vi "Check_Aero_Tunnel_on_Server.vi"(0 "Values":dbl[](array[numeric]) format="%.2f", 2 "Ch Names":string[](array[string]), 3 "Current Time":dbl format="%.2f", 4 "Adam Loop Count":i32) -> (6 "Scan comment":string)   [LabVIEW 2022 SP3]
uses:
  Controls/In_Range.ctl
  Aero Cooling Global.vi
panel:
  out "Tunnel Speed":dbl
  in  "Thermistor averaging length":i32=20
  out "Thermistor Temp":dbl format="%.2f"
  in  "Tweak time Down":dbl=100.0
  out "Reset Integral Term":bool
  in  "Tweak time Up":dbl=50.0
  in  "delta t per delta speed":dbl=0.3
  out "Significant speed change?":bool
  out "Valve Dem Pos":dbl
  out "Tweak in working section demanded temp":dbl
  out "Run Aero Chiller PID?":bool
  in  "Delta Speed greater than":dbl=5.0
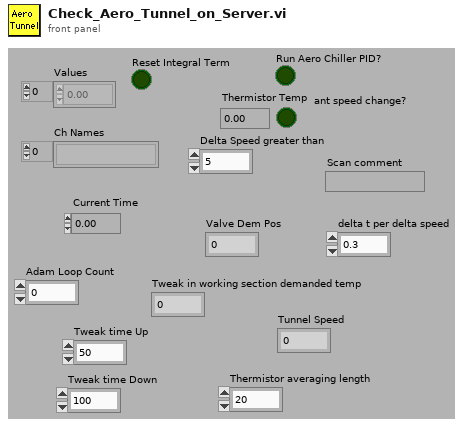
[diagram p1: front panel]
types:
  T1 = typedef "In_Range.ctl" = enum16{"%", "±", "% & ±"}
  T2 = typedef "LVDateTimeRec.ctl" = cluster{"fractional second":dbl, "second":i32, "minute":i32, "hour":i32, "day of month":i32, "month":i32, "year":i32, "day of week":i32, "day of year":i32, "DST":i32}
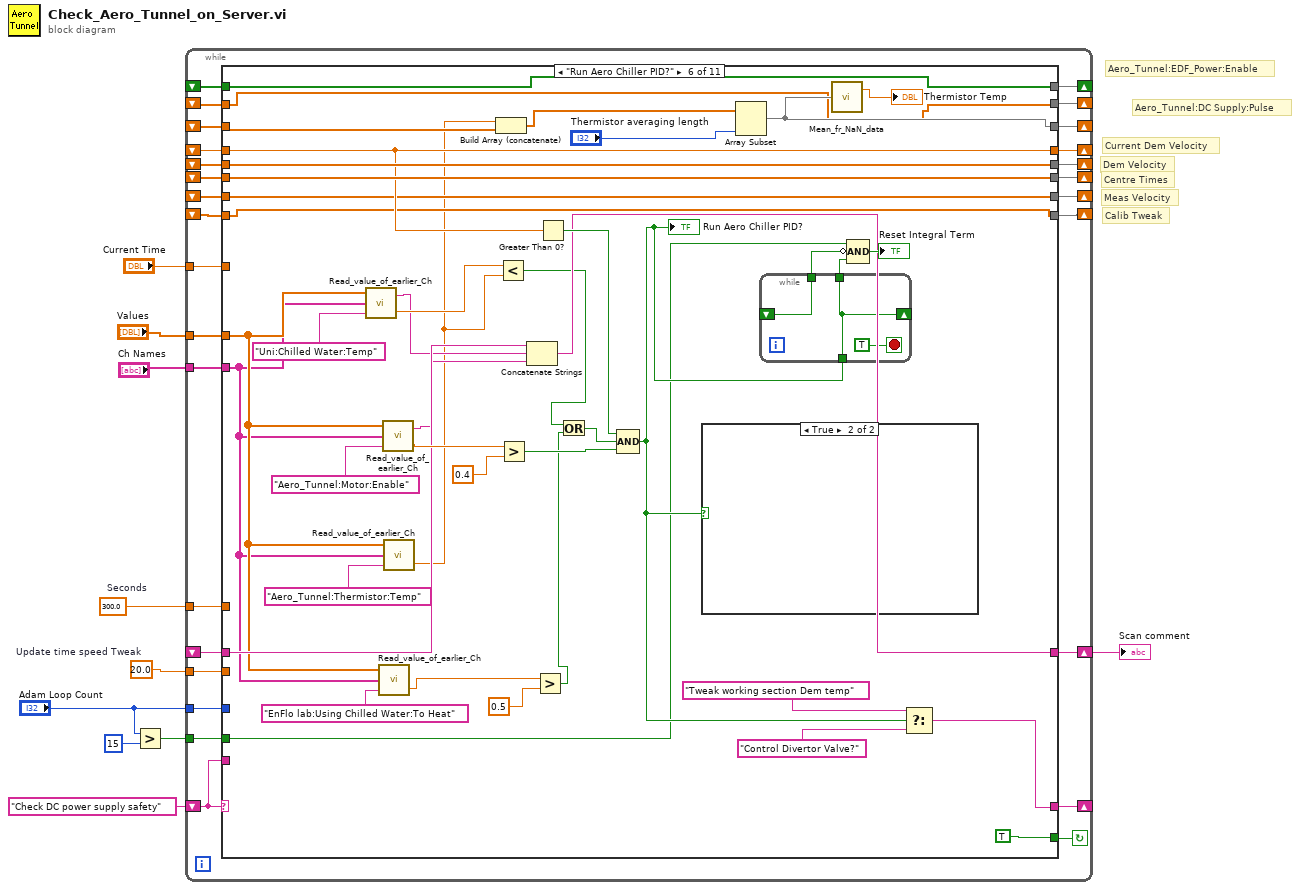
[diagram p0: block diagram]
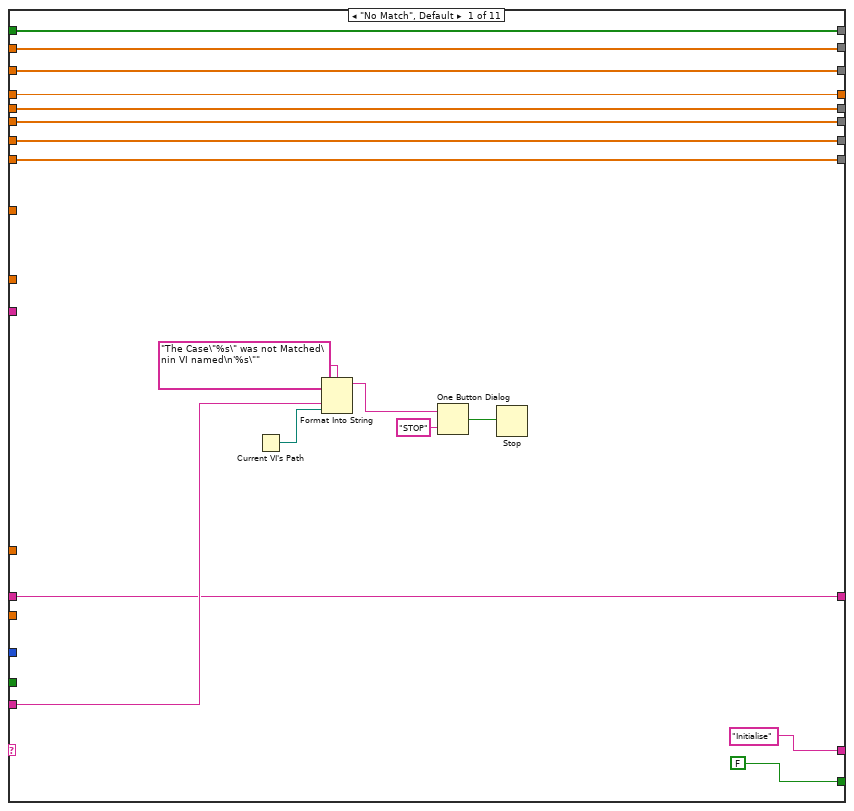
[diagram p2: hidden frame]
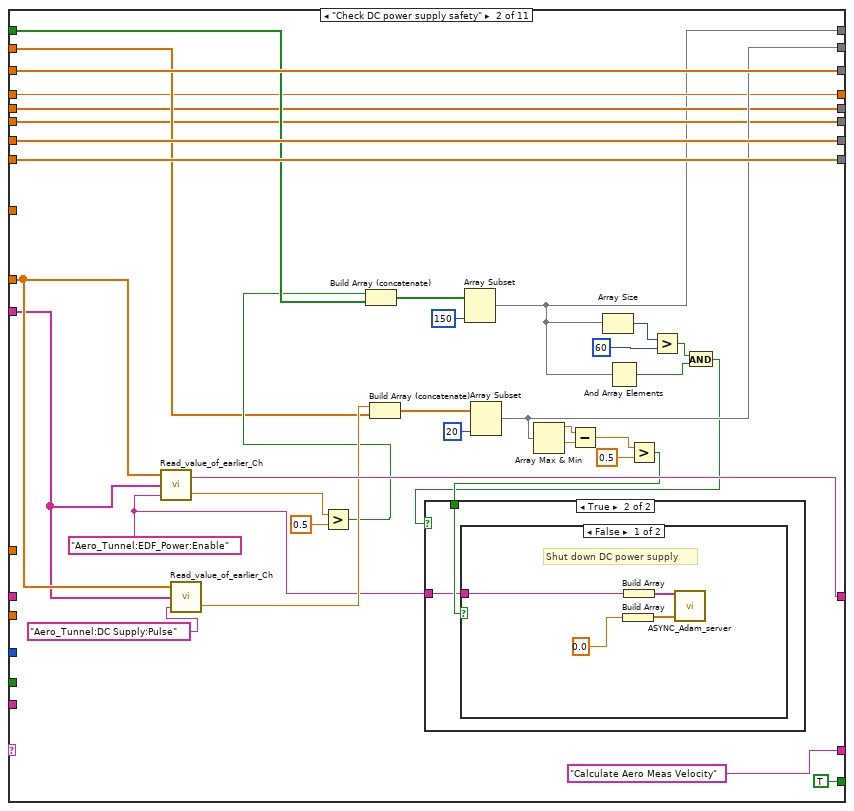
[diagram p3: hidden frame]
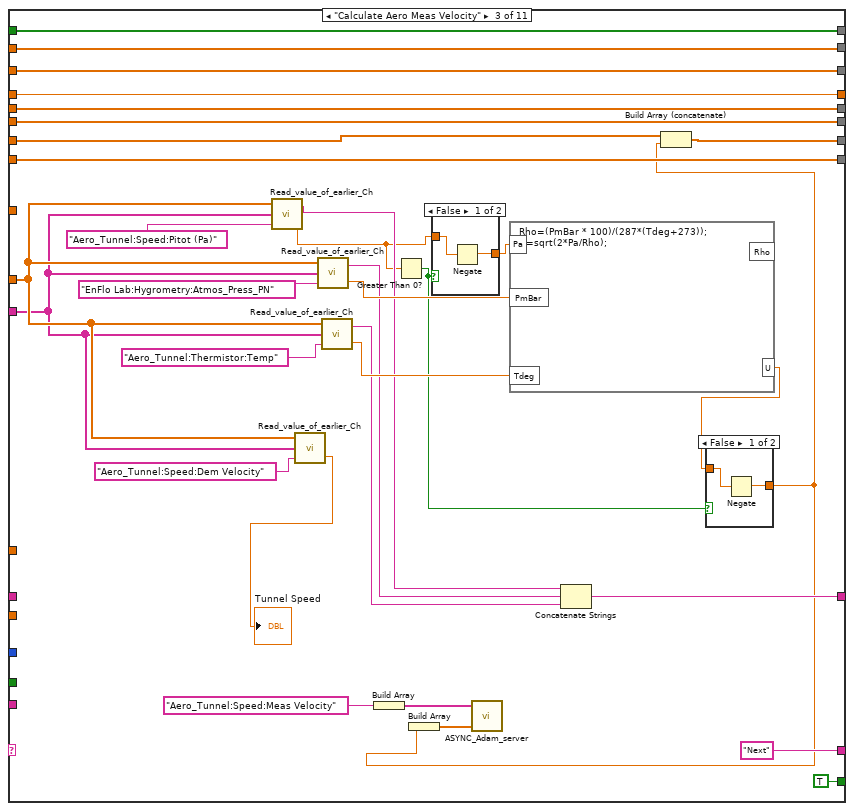
[diagram p6: hidden frame]
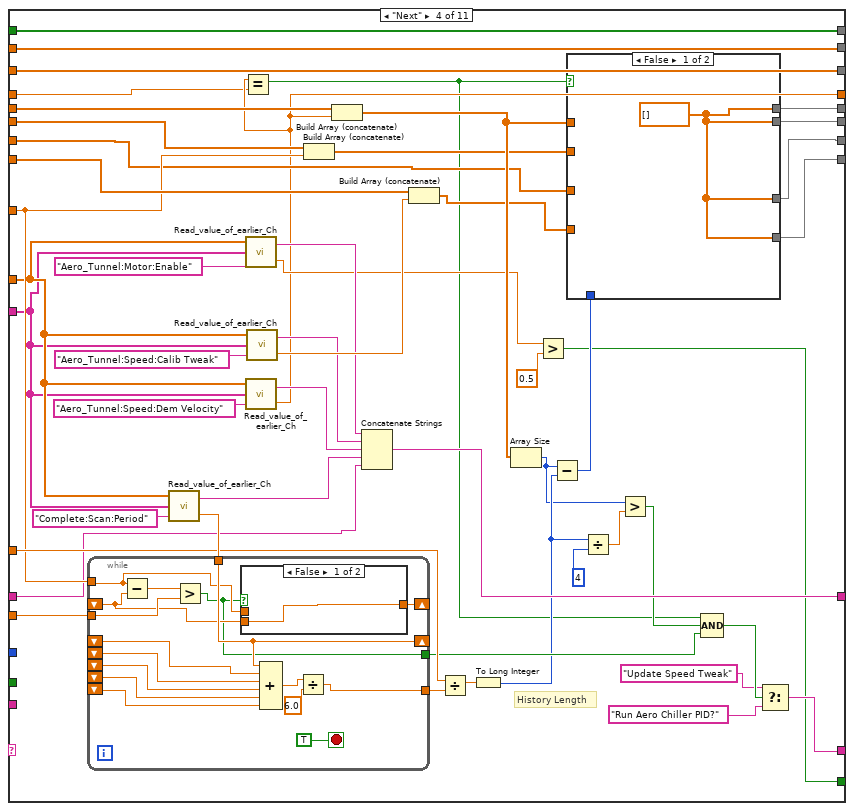
[diagram p9: hidden frame]
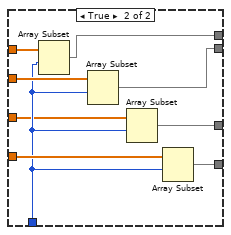
[diagram p10: hidden frame]
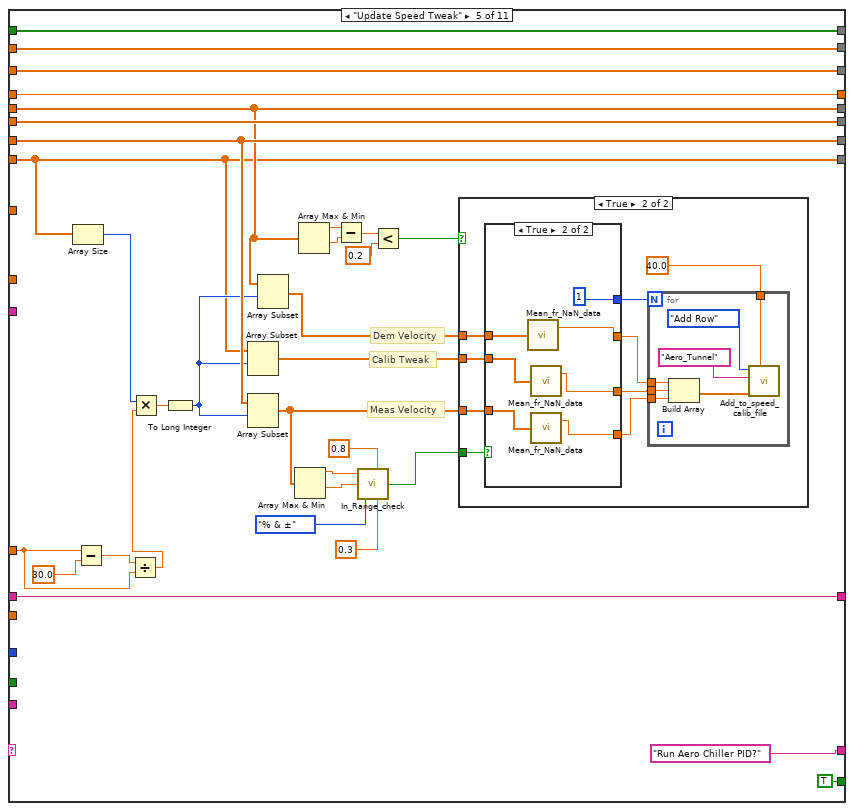
[diagram p12: hidden frame]
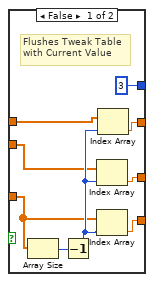
[diagram p14: hidden frame]
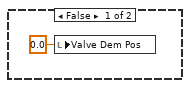
[diagram p15: hidden frame]
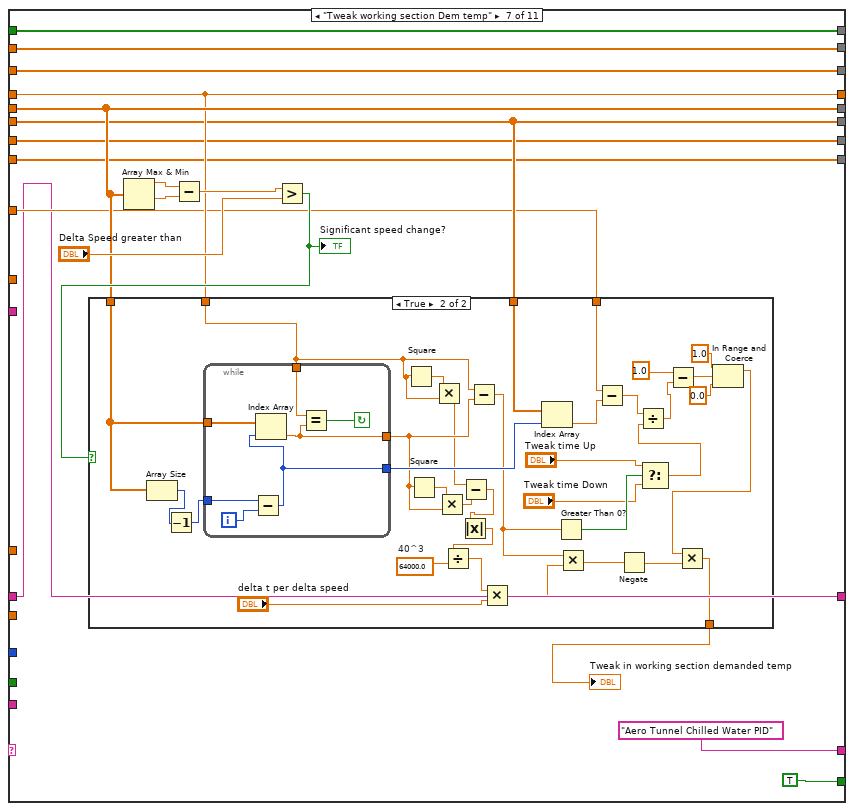
[diagram p16: hidden frame]
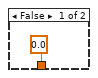
[diagram p17: hidden frame]
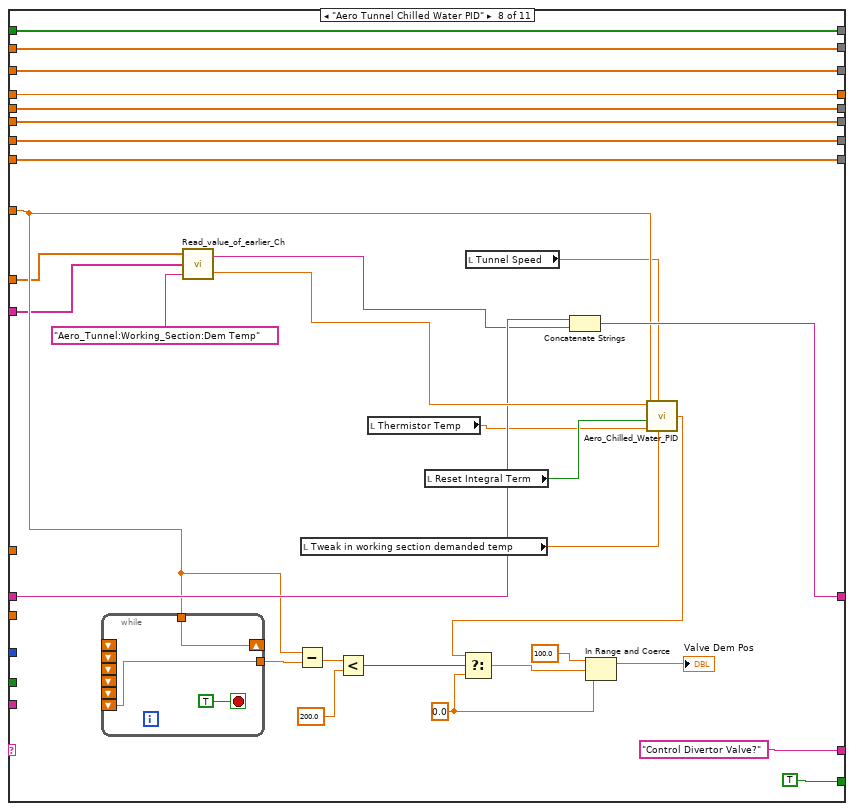
[diagram p18: hidden frame]
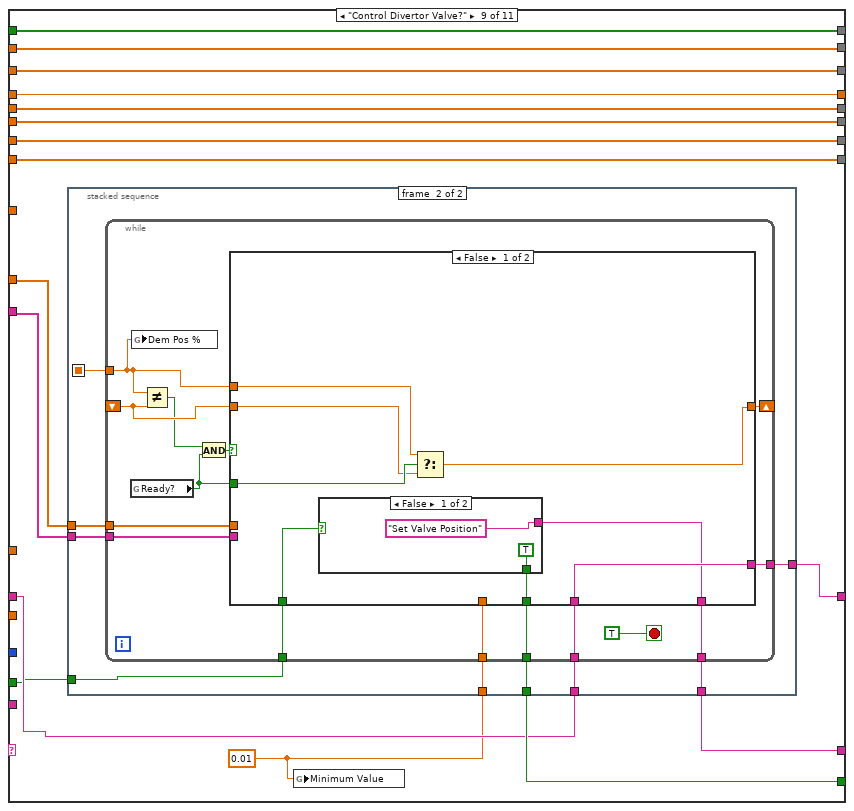
[diagram p19: hidden frame]
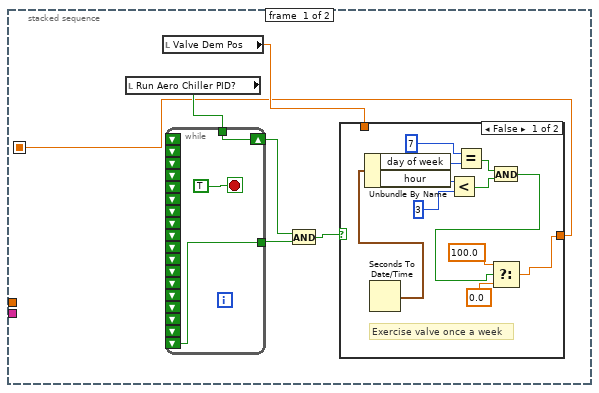
[diagram p20: hidden frame]
diagram:
  w3 = 20.0  # Update time speed Tweak
  w4 = 300.0  # Seconds
  # "Aero_Tunnel:DC Supply:Pulse"
  # "Aero_Tunnel:EDF_Power:Enable"
  # "Calib Tweak"
  # "Meas Velocity"
  # "Dem Velocity"
  # "Centre Times"
  # "Current Dem Velocity"
  n1 = Greater?(x="Adam Loop Count", y=15) -> (0:w6:bool)
  n2 = while {
    shift-left: "Check DC power supply safety" ("t") -> [w36]
    shift-right: [w37] -> _
    tunnel: "Values" -> [w35]
    tunnel: "Ch Names" -> [w34]
    shift-right: [w33] -> _
    shift-left: _ -> [w32]
    shift-right: [w30] -> _
    shift-left: _ -> [w31]
    shift-right: [w27] -> _
    shift-left: _ -> [w28]
    tunnel: "Current Time" -> [w29]
    tunnel: w6 -> [w26]
    shift-right: [w25] -> w5
    shift-left: _ -> [w24]
    tunnel: w4 -> [w23]
    shift-right: [w22] -> _
    shift-left: _ -> [w21]
    shift-right: [w20] -> _
    shift-left: _ -> [w19]
    tunnel: w3 -> [w18]
    tunnel: "Adam Loop Count" -> [w17]
    shift-right: [w15] -> _
    shift-left: _ -> [w16]
    shift-right: [w13] -> _
    shift-left: _ -> [w14]
    shift-right: [w11] -> _
    shift-left: _ -> [w12]
    stop <- w38 continue-if-true
    n3 = case shown="\"Run Aero Chiller PID?\"" w36 {
      tunnel: [FALSE TRUE TRUE w143 TRUE TRUE TRUE TRUE w422 FALSE FALSE] -> w38
      tunnel: ["Initialise" "Calculate Aero Meas Velocity" "Next" ("t") w158 "Run Aero Chiller PID?" ("t") w314 "Aero Tunnel Chilled Water PID" "Control Divertor Valve?" ("t") w419 "End" ("t") "End" ("t")] -> w37
      tunnel: w36 -> [w50 _ _ _ _ _ _ _ _ _ _]
      tunnel: w35 -> [_ w83 w99 w149 _ w284 _ w385 w424 _ _]
      tunnel: w34 -> [_ w82 w98 w148 _ w283 _ w384 w423 _ _]
      tunnel: [w47 w70 w123 w137 w243 w306 w332 w411 w430 w520 w564] -> w33
      tunnel: w32 -> [w47 w70 w123 w136 w243 w306 w332 w411 w430 w520 w564]
      tunnel: w31 -> [w46 w69 w122 w181 w219 w313 w333 w407 w432 w522 w566]
      tunnel: [w46 w69 w122 w179 w219 w313 w333 w407 w432 w522 w566] -> w30
      tunnel: w29 -> [_ _ _ w164 _ _ w330 w388 _ _ _]
      tunnel: w28 -> [w45 w68 w121 w177 w242 w312 w331 w412 w431 w521 w565]
      tunnel: [w45 w68 w121 w176 w242 w312 w331 w412 w431 w521 w565] -> w27
      tunnel: w26 -> [_ _ _ _ _ w301 _ _ w417 _ _]
      tunnel: [w44 w85 w111 w174 w241 w296 w328 w401 w420 w512 w550] -> w25
      tunnel: w24 -> [w44 _ _ w140 w241 w299 w328 w403 w421 w512 w552]
      tunnel: w23 -> [_ _ _ w173 w238 _ _ _ _ _ _]
      tunnel: [w43 w90 w124 w166 w231 w295 w327 w400 w429 w518 w562] -> w22
      tunnel: w21 -> [w43 w90 w127 w141 w231 w295 w327 w400 w429 w518 w562]
      tunnel: [w42 w89 w120 w165 w216 w294 w326 w399 w428 w517 w561] -> w20
      tunnel: w19 -> [w42 w89 w120 w168 w216 w294 w326 w399 w428 w517 w561]
      tunnel: w18 -> [_ _ _ w163 _ _ _ _ _ _ _]
      tunnel: w17 -> [_ _ _ _ _ _ _ _ _ _ _]
      tunnel: w16 -> [w41 w88 w126 w142 w218 w292 w325 w389 w427 w516 w560]
      tunnel: [w41 w88 w126 w142 w218 w288 w325 w389 w427 w516 w560] -> w15
      tunnel: w14 -> [w40 w80 w107 w139 w214 w286 w324 w387 w426 w515 w559]
      tunnel: [w40 w64 w107 w139 w214 w286 w324 w387 w426 w515 w559] -> w13
      tunnel: w12 -> [w39 w73 w106 w138 w213 w285 w323 w386 w425 w514 w558]
      tunnel: [w39 w72 w106 w138 w213 w285 w323 w386 w425 w514 w558] -> w11
      frame "No Match", Default {
        n4 = Current VI's Path() -> (path=w49:path)
        n5 = Format Into String(format string="The Case\"%s\" was not Matched\nin VI named\n'%s\"" ("Format String"), w50, w49) -> (resulting string=w53:string)  [unwired: 2 in, 1 out]
        n6 = One Button Dialog(message=w53, button name ("OK")="STOP") -> (true=w51:bool)
        n7 = Stop(stop? (T)=w51) -> ()
      }
      frame "Check DC power supply safety" {
        w65 = "Aero_Tunnel:EDF_Power:Enable" ("Desired Ch to Read")
        n8 = call "Read_value_of_earlier_Ch.vi"("Desired Ch to Read"=w65, "Ch names"=w82, "Present scan array"=w83) -> ("Value"=w81:dbl, "Scan comment"=w85:string)  [unwired: 1 in]
        n9 = call "Read_value_of_earlier_Ch.vi"("Desired Ch to Read"="Aero_Tunnel:DC Supply:Pulse", "Ch names"=w82, "Present scan array"=w83) -> ("Value"=w75:dbl)  [unwired: 1 in, 1 out]
        n10 = Greater?(x=w81, y=0.5) -> (0:w74:bool)
        n11 = Build Array (concatenate)(w74, w80) -> (w79:bool[])
        n12 = Build Array (concatenate)(w75, w73) -> (w76:dbl[])
        n13 = Array Subset(array=w79, length=150) -> (w64:bool[])  [unwired: 1 in]
        n14 = Array Subset(array=w76, length=20) -> (w72:dbl[])  [unwired: 1 in]
        n15 = Array Max & Min(array=w72) -> (max value=w58:dbl, min value=w57:dbl)  [unwired: 2 out]
        n16 = Subtract(x=w58, y=w57) -> (x-y=w56:dbl)
        n17 = Array Size(array=w64) -> (size(s)=w63:i32)
        n18 = And Array Elements(Boolean array=w64) -> (logical AND=w60:bool)
        n19 = Greater?(x=w56, y=0.5) -> (0:w66:bool)
        n20 = Greater?(x=w63, y=60) -> (0:w61:bool)
        n21 = And(x=w61, y=w60) -> (x .and. y?=w59:bool)
        n22 = case shown="True" w59 {
          tunnel: w66 -> [_ w92]
          tunnel: w65 -> [_ w91]
          frame False {
          }
          frame True {
            n23 = case shown="False" w92 {
              tunnel: w91 -> [w96 _]
              frame False {
                # "Shut down DC power supply"
                n24 = Build Array(0.0) -> (w94:dbl[])
                n25 = Build Array(w96) -> (w95:string[])
                n26 = call "ASYNC_Adam_server.vi"("Values"=w94, "Channel Names"=w95) -> ()  [unwired: 1 in, 3 out]
              }
              frame True {
              }
            }
          }
        }
      }
      frame "Calculate Aero Meas Velocity" {
        n27 = call "Read_value_of_earlier_Ch.vi"("Desired Ch to Read"="Aero_Tunnel:Speed:Pitot (Pa)", "Ch names"=w98, "Present scan array"=w99) -> ("Value"=w102:dbl, "Scan comment"=w114:string)  [unwired: 1 in]
        n28 = call "Read_value_of_earlier_Ch.vi"("Desired Ch to Read"="Aero_Tunnel:Speed:Dem Velocity", "Ch names"=w98, "Present scan array"=w99) -> ("Value"=→"Tunnel Speed":dbl)  [unwired: 1 in, 1 out]
        n29 = call "Read_value_of_earlier_Ch.vi"("Desired Ch to Read"="EnFlo Lab:Hygrometry:Atmos_Press_PN", "Ch names"=w98, "Present scan array"=w99) -> ("Value"=w116:dbl, "Scan comment"=w113:string)  [unwired: 1 in]
        n30 = call "Read_value_of_earlier_Ch.vi"("Desired Ch to Read"="Aero_Tunnel:Thermistor:Temp", "Ch names"=w98, "Present scan array"=w99) -> ("Value"=w115:dbl, "Scan comment"=w112:string)  [unwired: 1 in]
        n31 = Build Array("Aero_Tunnel:Speed:Meas Velocity") -> (w110:string[])
        n32 = Greater Than 0?(x=w102) -> (x > 0?=w103:bool)
        n33 = case shown="False" w103 {
          tunnel: [w132 w134] -> w101
          tunnel: w102 -> [w133 w134]
          frame False {
            n34 = Negate(x=w133) -> (-x=w132:dbl)
          }
          frame True {
          }
        }
        n35 = formula code="Rho=(PmBar * 100)/(287*(Tdeg+273));\nU=sqrt(2*Pa/Rho);"("Pa"=w101, "Tdeg"=w115, "PmBar"=w116) -> ("U"=w105:dbl)  [unwired: 1 out]
        n36 = Concatenate Strings(w114, w113, w112) -> (w111:string)
        n37 = case shown="False" w103 {
          tunnel: [w129 w131] -> w104
          tunnel: w105 -> [w130 w131]
          frame False {
            n38 = Negate(x=w130) -> (-x=w129:dbl)
          }
          frame True {
          }
        }
        n39 = Build Array(w104) -> (w109:dbl[])
        n40 = call "ASYNC_Adam_server.vi"("Values"=w109, "Channel Names"=w110) -> ()  [unwired: 1 in, 3 out]
        n41 = Build Array (concatenate)(w127, w104) -> (w124:dbl[])
      }
      frame "Next" {
        # "History Length"
        n42 = call "Read_value_of_earlier_Ch.vi"("Desired Ch to Read"="Complete:Scan:Period", "Ch names"=w148, "Present scan array"=w149) -> ("Value"=w183:dbl, "Scan comment"=w175:string)  [unwired: 1 in]
        n43 = while {
          shift-right: [w210] -> _
          shift-left: _ -> [w209]
          tunnel: w183 -> [w210]
          shift-left: _ -> [w208]
          shift-left: _ -> [w207]
          shift-left: _ -> [w206]
          shift-left: _ -> [w205]
          tunnel: [w201] -> w182
          tunnel: w164 -> [w197]
          shift-right: [w198] -> _
          shift-left: _ -> [w196]
          tunnel: w163 -> [w199]
          tunnel: [w195] -> w162
          stop <- TRUE stop-if-true
          n44 = Subtract(x=w197, y=w196) -> (x-y=w200:dbl)
          n45 = Greater?(x=w200, y=w199) -> (0:w195:bool)
          n46 = case shown="False" w195 {
            tunnel: [w211 w212] -> w198
            tunnel: w197 -> [_ w212]
            tunnel: w196 -> [w211 _]
            frame False {
            }
            frame True {
            }
          }
          n47 = Compound Arithmetic op=ADD(w210, w209, w208, w207, w206, w205) -> (w203:dbl)
          n48 = Divide(x=w203, y=6.0) -> (x/y=w201:dbl)
        }
        n49 = call "Read_value_of_earlier_Ch.vi"("Desired Ch to Read"="Aero_Tunnel:Motor:Enable", "Ch names"=w148, "Present scan array"=w149) -> ("Value"=w145:dbl, "Scan comment"=w146:string)  [unwired: 1 in]
        n50 = call "Read_value_of_earlier_Ch.vi"("Desired Ch to Read"="Aero_Tunnel:Speed:Dem Velocity", "Ch names"=w148, "Present scan array"=w149) -> ("Value"=w137:dbl, "Scan comment"=w156:string)  [unwired: 1 in]
        n51 = Equal?(x=w137, y=w136) -> (x = y?=w135:bool)
        n52 = call "Read_value_of_earlier_Ch.vi"("Desired Ch to Read"="Aero_Tunnel:Speed:Calib Tweak", "Ch names"=w148, "Present scan array"=w149) -> ("Value"=w169:dbl, "Scan comment"=w157:string)  [unwired: 1 in]
        n53 = Build Array (concatenate)(w177, w164) -> (w170:dbl[])
        n54 = Build Array (concatenate)(w181, w137) -> (w178:dbl[])
        n55 = Concatenate Strings(w146, w157, w156, w175, w140) -> (w174:string)
        n56 = Build Array (concatenate)(w168, w169) -> (w167:dbl[])
        n57 = Divide(x=w173, y=w182) -> (x/y=w180:dbl)
        n58 = To Long Integer(number=w180) -> (32bit integer=w154:i32)
        n59 = Array Size(array=w178) -> (size(s)=w153:i32)
        n60 = Greater?(x=w145, y=0.5) -> (0:w143:bool)
        n61 = Subtract(x=w153, y=w154) -> (x-y=w150:i32)
        n62 = case shown="False" w135 {
          tunnel: [w185 w194] -> w179
          tunnel: w178 -> [_ w193]
          tunnel: [w185 w192] -> w176
          tunnel: w170 -> [_ w191]
          tunnel: w167 -> [_ w190]
          tunnel: [w185 w189] -> w166
          tunnel: [w185 w188] -> w165
          tunnel: w150 -> [_ w187]
          tunnel: w141 -> [_ w186]
          frame False {
            w185 = dbl[] []
          }
          frame True {
            n63 = Array Subset(array=w193, index=w187) -> (w194:dbl[])  [unwired: 1 in]
            n64 = Array Subset(array=w191, index=w187) -> (w192:dbl[])  [unwired: 1 in]
            n65 = Array Subset(array=w186, index=w187) -> (w189:dbl[])  [unwired: 1 in]
            n66 = Array Subset(array=w190, index=w187) -> (w188:dbl[])  [unwired: 1 in]
          }
        }
        n67 = Divide(x=w154, y=4) -> (x/y=w152:dbl)
        n68 = Greater?(x=w153, y=w152) -> (0:w151:bool)
        n69 = Compound Arithmetic op=AND(w135, w151, w162) -> (w161:bool)
        n70 = Select(t="Update Speed Tweak", s=w161, f="Run Aero Chiller PID?" ("t")) -> (s? t:f=w158:string)
      }
      frame "Update Speed Tweak" {
        # "Meas Velocity"
        # "Calib Tweak"
        # "Dem Velocity"
        n71 = Array Size(array=w216) -> (size(s)=w215:i32)
        n72 = Subtract(x=w238, y=30.0) -> (x-y=w239:dbl)
        n73 = Divide(x=w239, y=w238) -> (x/y=w237:dbl)
        n74 = Multiply(x=w215, y=w237) -> (x*y=w236:dbl)
        n75 = To Long Integer(number=w236) -> (32bit integer=w229:i32)
        n76 = Array Subset(array=w216, index=w229) -> (w227:dbl[])  [unwired: 1 in]
        n77 = Array Subset(array=w231, index=w229) -> (w226:dbl[])  [unwired: 1 in]
        n78 = Array Subset(array=w219, index=w229) -> (w228:dbl[])  [unwired: 1 in]
        n79 = Array Max & Min(array=w226) -> (max value=w225:dbl, min value=w224:dbl)  [unwired: 2 out]
        n80 = Array Max & Min(array=w219) -> (max value=w235:dbl, min value=w234:dbl)  [unwired: 2 out]
        n81 = Subtract(x=w235, y=w234) -> (x-y=w233:dbl)
        n82 = call "In_Range_check.vi"("±"=0.3, "%"=0.8, "Mode"=In_Range."% & ±", "Value"=w224, "Setpoint"=w225) -> ("In Range"=w220:bool)  [unwired: 2 out]
        n83 = Less?(x=w233, y=0.2) -> (x < y?=w230:bool)
        n84 = case shown="True" w230 {
          tunnel: w228 -> [_ w253]
          tunnel: w227 -> [_ w252]
          tunnel: w226 -> [_ w251]
          tunnel: w220 -> [_ w247]
          frame False {
          }
          frame True {
            n85 = case shown="True" w247 {
              tunnel: w253 -> [w267 w276]
              tunnel: w252 -> [w266 w275]
              tunnel: w251 -> [w265 w274]
              tunnel: [w264 w273] -> w250
              tunnel: [w263 w272] -> w249
              tunnel: [w262 w271] -> w248
              tunnel: [3 1] -> w246
              frame False {
                # "Flushes Tweak Table\nwith Current Value"
                n86 = Array Size(array=w265) -> (size(s)=w269:i32)
                n87 = Decrement(x=w269) -> (x-1=w268:i32)
                n88 = Index Array(array=w266, index=w268) -> (element=w263:dbl)
                n89 = Index Array(array=w265, index=w268) -> (element=w264:dbl)
                n90 = Index Array(array=w267, index=w268) -> (element=w262:dbl)
              }
              frame True {
                n91 = call "Mean_fr_NaN_data.vi"("Data"=w276) -> ("Mean value"=w271:dbl)  [unwired: 1 out]
                n92 = call "Mean_fr_NaN_data.vi"("Data"=w275) -> ("Mean value"=w272:dbl)  [unwired: 1 out]
                n93 = call "Mean_fr_NaN_data.vi"("Data"=w274) -> ("Mean value"=w273:dbl)  [unwired: 1 out]
              }
            }
            n94 = for {
              N: w246 -> [_]
              tunnel: w250 -> [w257]
              tunnel: w249 -> [w256]
              tunnel: w248 -> [w255]
              tunnel: 40.0 ("Max Velocity") -> [w254]
              n95 = Build Array(w255, w256, w257) -> (w258:dbl[])
              n96 = call "Add_to_speed_calib_file.vi"("Max Velocity"=w254, "New Row"=w258, "Rig Name"="Aero_Tunnel" ("y"), "Mode"=enum16{"Add Row", "Get Error Value"}."Add Row") -> ()  [unwired: 2 in, 2 out]
            }
          }
        }
      }
      frame "Run Aero Chiller PID?" {
        n97 = call "Read_value_of_earlier_Ch.vi"("Desired Ch to Read"="Uni:Chilled Water:Temp", "Ch names"=w283, "Present scan array"=w284) -> ("Value"=w316:dbl, "Scan comment"=w298:string)  [unwired: 1 in]
        n98 = call "Read_value_of_earlier_Ch.vi"("Desired Ch to Read"="EnFlo lab:Using Chilled Water:To Heat", "Ch names"=w283, "Present scan array"=w284) -> ("Value"=w278:dbl)  [unwired: 1 in, 1 out]
        n99 = call "Read_value_of_earlier_Ch.vi"("Desired Ch to Read"="Aero_Tunnel:Motor:Enable", "Ch names"=w283, "Present scan array"=w284) -> ("Value"=w308:dbl, "Scan comment"=w297:string)  [unwired: 1 in]
        n100 = call "Read_value_of_earlier_Ch.vi"("Desired Ch to Read"="Aero_Tunnel:Thermistor:Temp", "Ch names"=w283, "Present scan array"=w284) -> ("Value"=w291:dbl)  [unwired: 1 in, 1 out]
        n101 = Build Array (concatenate)(w291, w292) -> (w290:dbl[])
        n102 = Less?(x=w316, y=w291) -> (x < y?=w281:bool)
        n103 = Greater?(x=w308, y=0.4) -> (0:w307:bool)
        n104 = Concatenate Strings(w299, w298, w297) -> (w296:string)
        n105 = Greater?(x=w278, y=0.5) -> (0:w277:bool)
        n106 = Greater Than 0?(x=w306) -> (x > 0?=w305:bool)
        n107 = Or(x=w281, y=w277) -> (x .or. y?=w280:bool)
        n108 = Compound Arithmetic op=AND(w305, w280, w307) -> (w304:bool)
        "Run Aero Chiller PID?" <- w304
        n109 = case shown="True" w304 {
          frame False {
            n110 = local write "Valve Dem Pos"(0.0 ("Valve Dem Pos")) -> ()
          }
          frame True {
          }
        }
        n111 = Array Subset(array=w290, length="Thermistor averaging length") -> (w288:dbl[])  [unwired: 1 in]
        n112 = while {
          shift-right: [w320] -> _
          shift-left: _ -> [w321]
          tunnel: w304 -> [w320]
          tunnel: [w321] -> w303
          tunnel: [w320] -> w302
          stop <- TRUE stop-if-true
        }
        n113 = call "Mean_fr_NaN_data.vi"("Data"=w288) -> ("Mean value"=→"Thermistor Temp":dbl)  [unwired: 1 out]
        n114 = Compound Arithmetic op=AND(w301, invert w303, w302) -> (→"Reset Integral Term":bool)
        n115 = Select(t="Tweak working section Dem temp", s=w304, f="Control Divertor Valve?") -> (s? t:f=w314:string)
      }
      frame "Tweak working section Dem temp" {
        n116 = Array Max & Min(array=w333) -> (max value=w337:dbl, min value=w338:dbl)  [unwired: 2 out]
        n117 = Subtract(x=w337, y=w338) -> (x-y=w336:dbl)
        n118 = Greater?(x=w336, y="Delta Speed greater than") -> (0:w334:bool)
        "Significant speed change?" <- w334
        n119 = case shown="True" w334 {
          tunnel: w333 -> [_ w374]
          tunnel: w332 -> [_ w348]
          tunnel: w331 -> [_ w371]
          tunnel: w330 -> [_ w370]
          tunnel: [0.0 w361] -> w329
          frame False {
          }
          frame True {
            w352 = 64000.0  # 40^3
            n120 = Array Size(array=w374) -> (size(s)=w373:i32)
            n121 = Decrement(x=w373) -> (x-1=w375:i32)
            n122 = while {
              tunnel: w375 -> [w381]
              tunnel: w374 -> [w380]
              tunnel: w348 -> [w379]
              tunnel: [w377] -> w372
              tunnel: [w376] -> w346
              i -> [w382]
              stop <- w378 continue-if-true
              n123 = Subtract(x=w381, y=w382) -> (x-y=w377:i32)
              n124 = Index Array(array=w380, index=w377) -> (element=w376:dbl)
              n125 = Equal?(x=w379, y=w376) -> (x = y?=w378:bool)
            }
            n126 = Square(x=w348) -> (x^2=w353:dbl)
            n127 = Square(x=w346) -> (x^2=w347:dbl)
            n128 = Multiply(x=w353, y=w348) -> (x*y=w344:dbl)
            n129 = Multiply(x=w347, y=w346) -> (x*y=w345:dbl)
            n130 = Subtract(x=w344, y=w345) -> (x-y=w343:dbl)
            n131 = Absolute Value(x=w343) -> (abs(x)=w342:dbl)
            n132 = Divide(x=w342, y=w352) -> (x/y=w351:dbl)
            n133 = Subtract(x=w348, y=w346) -> (x-y=w358:dbl)
            n134 = Multiply(x=w351, y="delta t per delta speed") -> (x*y=w349:dbl)
            n135 = Index Array(array=w371, index=w372) -> (element=w369:dbl)
            n136 = Greater Than 0?(x=w358) -> (x > 0?=w357:bool)
            n137 = Multiply(x=w358, y=w349) -> (x*y=w360:dbl)
            n138 = Subtract(x=w370, y=w369) -> (x-y=w367:dbl)
            n139 = Negate(x=w360) -> (-x=w359:dbl)
            n140 = Select(t="Tweak time Up", s=w357, f="Tweak time Down") -> (s? t:f=w354:dbl)
            n141 = Divide(x=w367, y=w354) -> (x/y=w366:dbl)
            n142 = Subtract(x=1.0, y=w366) -> (x-y=w365:dbl)
            n143 = In Range and Coerce(upper limit=1.0, x=w365, lower limit=0.0) -> (coerced(x)=w362:dbl)  [unwired: 1 out]
            n144 = Multiply(x=w362, y=w359) -> (x*y=w361:dbl)
          }
        }
        "Tweak in working section demanded temp" <- w329
      }
      frame "Aero Tunnel Chilled Water PID" {
        w392 = 0.0 ("lower limit")
        n145 = while {
          shift-right: [w416] -> _
          shift-left: _ -> [_]
          tunnel: w388 -> [w416]
          shift-left: _ -> [_]
          shift-left: _ -> [_]
          shift-left: _ -> [_]
          shift-left: _ -> [_]
          shift-left: _ -> [w415]
          tunnel: [w415] -> w397
          stop <- TRUE stop-if-true
        }
        n146 = call "Read_value_of_earlier_Ch.vi"("Desired Ch to Read"="Aero_Tunnel:Working_Section:Dem Temp", "Ch names"=w384, "Present scan array"=w385) -> ("Value"=w404:dbl, "Scan comment"=w402:string)  [unwired: 1 in]
        n147 = Subtract(x=w388, y=w397) -> (x-y=w396:dbl)
        n148 = local read "Tweak in working section demanded temp"() -> (w405:dbl)
        n149 = Less?(x=w396, y=200.0) -> (x < y?=w394:bool)
        n150 = local read "Thermistor Temp"() -> (w390:dbl)
        n151 = local read "Reset Integral Term"() -> (w406:bool)
        n152 = local read "Tunnel Speed"() -> (w383:dbl)
        n153 = Concatenate Strings(w403, w402) -> (w401:string)
        n154 = call "Aero_Chilled_Water_PID.vi"("Tweak in working section demanded temp"=w405, "Tunnel Speed"=w383, "Present Value"=w390, "Reset PID"=w406, "Current Time"=w388, "Setpoint"=w404) -> ("Dem Output"=w393:dbl)
        n155 = Select(t=w393, s=w394, f=w392) -> (s? t:f=w391:dbl)
        n156 = In Range and Coerce(upper limit=100.0, x=w391, lower limit=w392) -> (coerced(x)=→"Valve Dem Pos":dbl)  [unwired: 1 out]
      }
      frame "Control Divertor Valve?" {
        w418 = 0.01 ("lower limit")
        n157 = stacked-sequence {
          seq-local: [w433 _] -> [_ w462]
          tunnel: w424 -> [_ w461]
          tunnel: w423 -> [_ w460]
          tunnel: [_ w459] -> w422
          tunnel: w421 -> [_ w458]
          tunnel: [_ w457] -> w420
          tunnel: [_ w456] -> w419
          tunnel: w418 -> [_ w455]
          tunnel: w417 -> [_ w454]
          frame #0 {
            n158 = local read "Run Aero Chiller PID?"() -> (w435:bool)
            n159 = local read "Valve Dem Pos"() -> (w434:dbl)
            n160 = while {
              shift-right: [w453] -> w436
              shift-left: _ -> [_]
              tunnel: w435 -> [w453]
              shift-left: _ -> [_]
              shift-left: _ -> [_]
              shift-left: _ -> [_]
              shift-left: _ -> [_]
              shift-left: _ -> [_]
              shift-left: _ -> [_]
              shift-left: _ -> [_]
              shift-left: _ -> [_]
              shift-left: _ -> [_]
              shift-left: _ -> [_]
              shift-left: _ -> [_]
              shift-left: _ -> [_]
              shift-left: _ -> [_]
              shift-left: _ -> [_]
              shift-left: _ -> [_]
              shift-left: _ -> [_]
              shift-left: _ -> [w452]
              tunnel: [w452] -> w437
              stop <- TRUE stop-if-true
            }
            n161 = And(x=w436, y=w437) -> (x .and. y?=w438:bool)
            n162 = case shown="False" w438 {
              tunnel: [w440 w450] -> w433
              tunnel: w434 -> [_ w450]
              frame False {
                # "Exercise valve once a week"
                n163 = Seconds To Date/Time() -> (date time rec=w441:T2)  [unwired: 2 out]
                n164 = Unbundle By Name(w441) -> ("day of week"=w446:i32, "hour"=w444:i32)
                n165 = Less?(x=w444, y=3) -> (x < y?=w449:bool)
                n166 = Equal?(x=7, y=w446) -> (x = y?=w448:bool)
                n167 = And(x=w448, y=w449) -> (x .and. y?=w439:bool)
                n168 = Select(t=100.0, s=w439, f=0.0) -> (s? t:f=w440:dbl)
              }
              frame True {
              }
            }
          }
          frame #1 {
            n169 = while {
              shift-right: [w469] -> _
              shift-left: _ -> [w468]
              tunnel: w462 -> [w466]
              tunnel: w461 -> [w476]
              tunnel: w460 -> [w475]
              tunnel: [w474] -> w459
              tunnel: w458 -> [w473]
              tunnel: [w472] -> w457
              tunnel: [w471] -> w456
              tunnel: w455 -> [w464]
              tunnel: w454 -> [w463]
              stop <- TRUE stop-if-true
              n170 = global read "Aero Cooling Global.vi" "Ready?"() -> (w465:bool)
              n171 = global write "Aero Cooling Global.vi" "Dem Pos %"(w466) -> ()
              n172 = Not Equal?(x=w466, y=w468) -> (x != y?=w467:bool)
              n173 = And(x=w467, y=w465) -> (x .and. y?=w470:bool)
              n174 = case shown="False" w470 {
                tunnel: w476 -> [_ w507]
                tunnel: w475 -> [_ w506]
                tunnel: [w479 TRUE] -> w474
                tunnel: w473 -> [w485 w503]
                tunnel: [w485 w502] -> w472
                tunnel: [w478 w496] -> w471
                tunnel: [w482 w491] -> w469
                tunnel: w466 -> [w483 w493]
                tunnel: w468 -> [w481 w494]
                tunnel: w465 -> [w484 _]
                tunnel: w464 -> [_ w490]
                tunnel: w463 -> [w480 _]
                frame False {
                  n175 = case shown="False" w480 {
                    tunnel: [TRUE FALSE] -> w479
                    tunnel: ["Set Valve Position" ("t") "End" ("t")] -> w478
                    frame False {
                    }
                    frame True {
                    }
                  }
                  n176 = Select(t=w483, s=w484, f=w481) -> (s? t:f=w482:dbl)
                }
                frame True {
                  n177 = call "Read_value_of_earlier_Ch.vi"("Desired Ch to Read"="Aero_Tunnel:Cooling_Div_Valve:Meas Pos", "Ch names"=w506, "Present scan array"=w507) -> ("Value"=w500:dbl, "Scan comment"=w501:string)  [unwired: 1 in]
                  n178 = Subtract(x=w493, y=w494) -> (x-y=w499:dbl)
                  n179 = global write "Aero Cooling Global.vi" "Meas Pos %"(w500) -> ()
                  n180 = Absolute Value(x=w499) -> (abs(x)=w492:dbl)
                  n181 = Less?(x=w492, y=w490) -> (x < y?=w495:bool)
                  n182 = Select(t=w494, s=w495, f=w493) -> (s? t:f=w491:dbl)
                  n183 = In Range and Coerce(upper limit=4.0, x=w492, lower limit=w490) -> (In Range?=w497:bool)  [unwired: 1 out]
                  n184 = case shown="False" w497 {
                    tunnel: ["Set Valve Position" ("t") "Async Control" ("t")] -> w496
                    frame False {
                    }
                    frame True {
                      n185 = global write "Aero Cooling Global.vi" "Ready?"(FALSE ("Ready?")) -> ()
                    }
                  }
                  n186 = Concatenate Strings(w503, w501) -> (w502:string)
                }
              }
            }
          }
        }
        n187 = global write "Aero Cooling Global.vi" "Minimum Value"(w418) -> ()
      }
      frame "Async Control" {
        n188 = while {
          shift-right: [w526] -> _
          shift-left: _ -> [w525]
          shift-right: [w523] -> _
          shift-left: TRUE -> [w527]
          stop <- w524 continue-if-true
          n189 = case shown="True" w527 {
            tunnel: [w532 w538] -> w526
            tunnel: w525 -> [w531 _]
            tunnel: [w529 FALSE ("status")] -> w524
            tunnel: [FALSE FALSE] -> w523
            frame True {
              n190 = invoke class="VI" method="Run VI"(reference=w531, "Wait until done"=FALSE ("Wait Until Done"), "Auto Dispose Ref"=TRUE) -> (reference out=w532:refnum<vi>, error out=w530:errorcluster)  [unwired: 2 in, 3 out]
              n191 = Unbundle By Name(w530) -> ("status"=w529:bool)
            }
            frame False {
              w540 = "Aero Cooling Valve Async.vi"
              w548 = FALSE  # Dialog Box (T)
              n192 = Current VI's Path() -> (path=w542:path)
              n193 = Strip Path(path=w542) -> (stripped path=w541:path)  [unwired: 1 out]
              n194 = Build Path(base path=w541, name or relative path=w540) -> (appended path=w539:path)
              n195 = Open VI Reference(vi path=w539) -> (vi reference=w545:refnum<vi>, error out=w544:errorcluster)  [unwired: 2 in, 3 out]
              n196 = invoke class="VI" method="Run VI"(reference=w545, error in=w544, "Wait until done"=FALSE ("Wait Until Done"), "Auto Dispose Ref"=TRUE) -> (reference out=w538:refnum<vi>, error out=w537:errorcluster)  [unwired: 1 in, 3 out]
              n197 = Concatenate Strings("Launching " ("Error Type"), w540) -> (w546:string)
              n198 = call "EnFlo_Error_Handler.vi"("error in (no error)"=w537, "Error Type"=w546, "Dialog Box (F)"=w548) -> ()  [unwired: 3 out]
            }
          }
        }
      }
      frame "Set Valve Position" {
        n199 = global read "Aero Cooling Global.vi" "Dem Pos %"() -> (w553:dbl)
        n200 = Build Array("Aero_Tunnel:Cooling_Div_Valve:Dem Pos") -> (w556:string[])
        n201 = Build Array(w553) -> (w554:dbl[])
        n202 = call "ASYNC_Adam_server.vi"("Values"=w554, "Channel Names"=w556) -> ("Scan Comments"=w551:string[])  [unwired: 2 in, 1 out]
        n203 = Concatenate Strings(w552, w551) -> (w550:string)
      }
    }
  }
  "Scan comment" <- w5
